vi "Process Data.vi"(7 "AdasLvTemplate in":refnum<class "AdasLvTemplate.lvclass">, 8 "error in":errorcluster, 11 "Node in":refnum<class "AMS Cycler Template.lvclass">) -> (0 "error out":errorcluster, 3 "Node out":refnum<class "AMS Cycler Template.lvclass">, 5 "AdasLvTemplate out":refnum<class "AdasLvTemplate.lvclass">)   [LabVIEW 2023, in "AMS Cycler Template.lvlib" / "AMS Cycler Template.lvclass"]
uses:
  AMS Cycler Template.lvclass
  <vilib>/ADAS Replay HIL/ADAS Plugin Utilities/AdasLvTemplate/AdasLvTemplate.lvclass
  AMS Cycler Template.lvclass/AMS Cycler Template.ctl
  C:/Program Files/National Instruments/AMS plugin/Capabilities/Capabilities/High Level Capabilities/Cycler Cluster/Cycler Cluster.lvclass
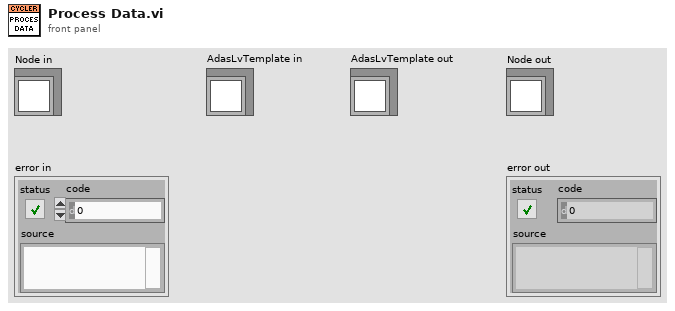
[diagram p1: front panel]
types:
  T1 = typedef "Cycler Cluster.lvclass/Consumer Ch.ctl" = cluster{"ErrorAcknowledge.ACT":bool, "OutputEnable.ACT":bool, "ControlMode.CTL":u16, "Voltage.SP":dbl, "VoltageMIN.SP":dbl, "VoltageMAX.SP":dbl, "VoltageGrad.SP":dbl, "Current.SP":dbl, "CurrentMIN.SP":dbl, "CurrentMAX.SP":dbl, "CurrentGrad.SP":dbl, "Power.SP":dbl, "PowerMIN.SP":dbl, "PowerMAX.SP":dbl, "PowerGrad.SP":dbl, "ParameterSet.CTL":i32}
  T2 = typedef "Cycler Cluster.lvclass/Consumer Control.ctl" = cluster{"OnOff.ACT":bool, "ErrorAcknowledge.ACT":bool, "IsoMeasurement.ACT":bool, "ParallelMode.ACT":bool}
  T3 = cluster{"Error.STS":i32, "OutputEnable.STS":i32, "ControlMode.STS":u16, "Voltage.AV":dbl, "Current.AV":dbl, "Power.AV":dbl, "VoltageNominal.AV":dbl, "CurrentNominal.AV":dbl, "PowerNominal.AV":dbl, "ParameterSet.STS":i32}[]
  T4 = typedef "Cycler Cluster.lvclass/Producer Control.ctl" = cluster{"OnOff.STS":i32, "Error.STS":i32, "Watchdog.STS":i32, "IsoMeasurement.STS":i32, "ParallelMode.STS":i32}
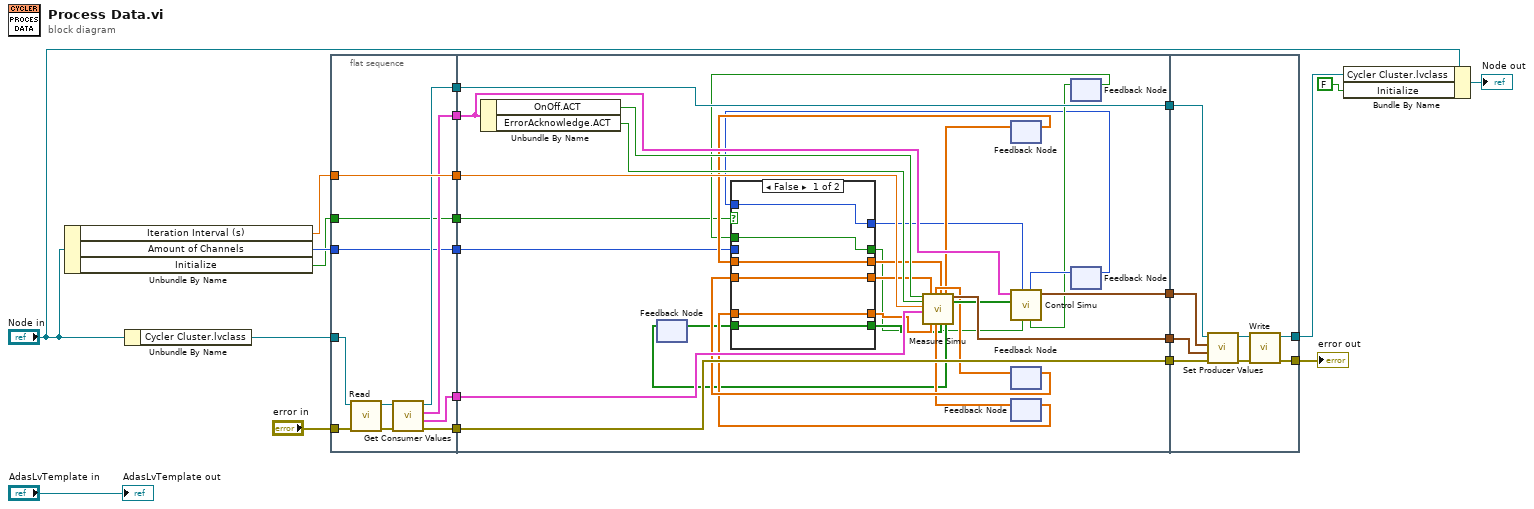
[diagram p0: block diagram]
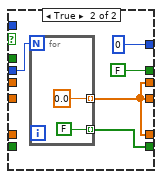
[diagram p2: hidden frame]
diagram:
  n1 = Unbundle By Name("Node in") -> ("Iteration Interval (s)"=w15:dbl, "Amount of Channels"=w4:u32, "Initialize"=w2:bool)
  n2 = Unbundle By Name("Node in") -> ("Cycler Cluster.lvclass"=w21:refnum<class "Cycler Cluster.lvclass">)
  n3 = flat-sequence {
    tunnel: w21 -> [w33]
    tunnel: "error in" -> [w32]
    tunnel: [w28] -> w13
    tunnel: [w26] -> w12
    tunnel: w15 -> [w31]
    tunnel: [w31] -> w11
    tunnel: [w27] -> w10
    tunnel: [w25] -> w9
    tunnel: w4 -> [w24]
    tunnel: [w24] -> w3
    tunnel: w2 -> [w23]
    tunnel: [w23] -> w1
    tunnel: w13 -> [w63]
    tunnel: [w63] -> w8
    tunnel: [w62] -> w7
    tunnel: [w61] -> w6
    tunnel: w12 -> [w60]
    tunnel: [w60] -> w5
    tunnel: w11 -> [w59]
    tunnel: w10 -> [w54]
    tunnel: w9 -> [w58]
    tunnel: w3 -> [w36]
    tunnel: w1 -> [w35]
    tunnel: [w84] -> w19
    tunnel: w8 -> [w82]
    tunnel: [w83] -> w16
    tunnel: w7 -> [w78]
    tunnel: w6 -> [w77]
    tunnel: w5 -> [w79]
    frame #0 {
      n4 = call-dynamic "Read.vi"("error in"=w32, "Cycler Cluster.lvclass in"=w33) -> ("error out"=w29:errorcluster, "Cycler Cluster.lvclass out"=w30:refnum<class "Cycler Cluster.lvclass">)  [unwired: 8 in]
      n5 = call "Get Consumer Values.vi"("error in"=w29, "Cycler Cluster.lvclass in"=w30) -> ("error out"=w28:errorcluster, "Consumer Ch"=w25:T1[], "Consumer Control"=w27:T2, "Cycler Cluster.lvclass out"=w26:refnum<class "Cycler Cluster.lvclass">)  [unwired: 6 in]
    }
    frame #1 {
      n6 = Unbundle By Name(w54) -> ("OnOff.ACT"=w57:bool, "ErrorAcknowledge.ACT"=w56:bool)
      n7 = feedback #1() -> (w42:bool[])  [unwired: 1 in]
      n8 = feedback #2() -> (w51:dbl[])  [unwired: 1 in]
      n9 = feedback #3() -> (w48:dbl[])  [unwired: 1 in]
      n10 = feedback #4() -> (w47:dbl[])  [unwired: 1 in]
      n11 = feedback #5() -> (w38:bool)  [unwired: 1 in]
      n12 = feedback #6() -> (w34:i32)  [unwired: 1 in]
      n13 = case shown="False" w35 {
        tunnel: w36 -> [_ w74]
        tunnel: [w64 FALSE ("Error Feedback out")] -> w37
        tunnel: [w66 w72] -> w44
        tunnel: w51 -> [w69 _]
        tunnel: [w69 w71] -> w50
        tunnel: w48 -> [w68 _]
        tunnel: [w68 w71] -> w49
        tunnel: w47 -> [w67 _]
        tunnel: [w67 w71] -> w46
        tunnel: w42 -> [w66 _]
        tunnel: w34 -> [w65 _]
        tunnel: [w65 0 ("Watchdog Feedback Out")] -> w40
        tunnel: w38 -> [w64 _]
        frame False {
        }
        frame True {
          n14 = for {
            N: w74 -> [_]
            tunnel: [0.0 ("Current Setpoint")] -> w71 mode=indexing
            tunnel: [FALSE ("Feedback Out")] -> w72 mode=indexing
          }
        }
      }
      n15 = call "Measure Simu.vi"("OnOff.ACT"=w57, "ErrorAcknowledge.ACT"=w56, "Iteration Interval (s)"=w59, "Channels In"=w58, "Current Feedback In"=w49, "Voltage Feedback In"=w46, "Power Feedback In"=w50, "Error Feedback In"=w44) -> ("Current Feedback Out"=w53:dbl[], "Voltage Feedback Out"=w45:dbl[], "Power Feedback out"=w52:dbl[], "Error Feedback Out"=w43:bool[], "Channels Out"=w61:T3, "Error Out"=w55:bool[])  [unwired: 6 in]
      n16 = feedback-in #1(w43) -> ()
      n17 = feedback-in #2(w52) -> ()
      n18 = call "Control Simu.vi"("Error Feedback"=w37, "Watchdog Feedback In"=w40, "Error Ch"=w55, "Controls In"=w54) -> ("Controls Out"=w62:T4, "Error Feedback out"=w39:bool, "Watchdog Feedback Out"=w41:i32)  [unwired: 5 in]
      n19 = feedback-in #3(w53) -> ()
      n20 = feedback-in #4(w45) -> ()
      n21 = feedback-in #5(w39) -> ()
      n22 = feedback-in #6(w41) -> ()
    }
    frame #2 {
      n23 = call "Set Producer Values.vi"("error in"=w82, "Producer Ch"=w77, "Producer Control"=w78, "Cycler Cluster.lvclass in"=w79) -> ("error out"=w81:errorcluster, "Cycler Cluster.lvclass out"=w80:refnum<class "Cycler Cluster.lvclass">)  [unwired: 6 in]
      n24 = call-dynamic "Write.vi"("error in"=w81, "Cycler Cluster.lvclass in"=w80) -> ("error out"=w83:errorcluster, "Cycler Cluster.lvclass out"=w84:refnum<class "Cycler Cluster.lvclass">)  [unwired: 8 in]
    }
  }
  n25 = Bundle By Name(cluster="Node in", "Cycler Cluster.lvclass"=w19, "Initialize"=FALSE) -> (→"Node out":refnum<class "AMS Cycler Template.lvclass">)
  "error out" <- w16
  "AdasLvTemplate out" <- "AdasLvTemplate in"
